vi "IMAGENES_SUB0.vi"() -> ()   [LabVIEW 2016]
uses:
  <vilib>/imath/engines/lvmath2/RunTimeEngine/BuiltInFunctions/round/NIMS_round(DBL-S).vi
  <vilib>/imath/engines/lvmath2/RunTimeEngine/NodeEndStatement/NIMS_NodeEndStatement_Output.vi
  <instcachedir>/0/NIMS_NodeEndStatement_Output_53EC0D466D134D7ABD903AC30B43404B.lvgen/NIMS_NodeEndStatement_Output_53EC0D466D134D7ABD903AC30B43404B_010.vi
  <vilib>/imath/engines/lvmath2/RunTimeEngine/ErrorHandling/NIMS_Finalize Error.vi
  <instcachedir>/0/NIMS_NodeEndStatement_Output_53EC0D466D134D7ABD903AC30B43404B.lvgen/NIMS_NodeEndStatement_Output_53EC0D466D134D7ABD903AC30B43404B_001.vi
  <vilib>/imath/engines/lvmath2/RunTimeEngine/RangeToken/NIMS_Range_R3 - Integer.vi
  <instcachedir>/0/NIMS_Range_R3 - Integer_A435E2FF893B4C718FD5055FE39FE2F6.lvgen/NIMS_Range_R3 - Integer_A435E2FF893B4C718FD5055FE39FE2F6_000.vi
  <vilib>/imath/engines/lvmath2/RunTimeEngine/CommandStatement/MC_CommandStatement_break.vi
  <vilib>/imath/engines/lvmath2/RunTimeEngine/VariableToken/NIMS_VariableToken_CondDefinedDefinedByReplace.vi
  <instcachedir>/0/NIMS_VariableToken_CondDefinedDefinedByReplace_D162CFFC24174562A9FEA619A91E1A56.lvgen/NIMS_VariableToken_CondDefinedDefinedByReplace_D162CFFC24174562A9FEA619A91E1A56_001.vi
  <vilib>/imath/engines/lvmath2/RunTimeEngine/IndexReplace/NIMS M(S,S)=S.vi
  <instcachedir>/0/NIMS M(S,S)=S_98E40400474E4398B113AE20298B4F82.lvgen/NIMS M(S,S)=S_98E40400474E4398B113AE20298B4F82_000.vi
  <vilib>/imathl/engines/lvmath/Functions/Error Handling/Create Error.vi
  <vilib>/imath/engines/lvmath2/RunTimeEngine/VariableToken/NIMS_VariableToken_CondDefined.vi
  <instcachedir>/0/NIMS_VariableToken_CondDefined_06E9DA95BD4D46A6BA55EC651A891960.lvgen/NIMS_VariableToken_CondDefined_06E9DA95BD4D46A6BA55EC651A891960_001.vi
  <vilib>/imath/engines/lvmath/Functions/Error Handling/MergeErrorsWrapper.vi
  <instcachedir>/0/NIMS_NodeEndStatement_Output_53EC0D466D134D7ABD903AC30B43404B.lvgen/NIMS_NodeEndStatement_Output_53EC0D466D134D7ABD903AC30B43404B_012.vi
panel:
  out "Anchura 2":i32
  out "Altura 2":i32
  out "Color":u32(colorbox)
  out "Anchura":i32
  out "Altura":i32
  out "IMAGEN_ORIGINAL":picture
  out "IMAGEN_MODIFICADA":picture
  out "Waveform Graph":dbl[](graph)
  in  "IMAGEN 1":path
  in  "Enum":T1(ring)
  in  "ZOOM":dbl(slide) min=0.1 max=10.0 step=0.01 scale=0.1..10.0
  in  "Desplazamiento X":dbl(slide) min=-500.0 max=500.0 step=1.0 scale=-500.0..500.0
  in  "Desplazamiento Y":dbl(slide)=500.0 min=-500.0 max=500.0 step=1.0 scale=-500.0..500.0
  in  "Giro":dbl(knob) scale=-360.0..360.0
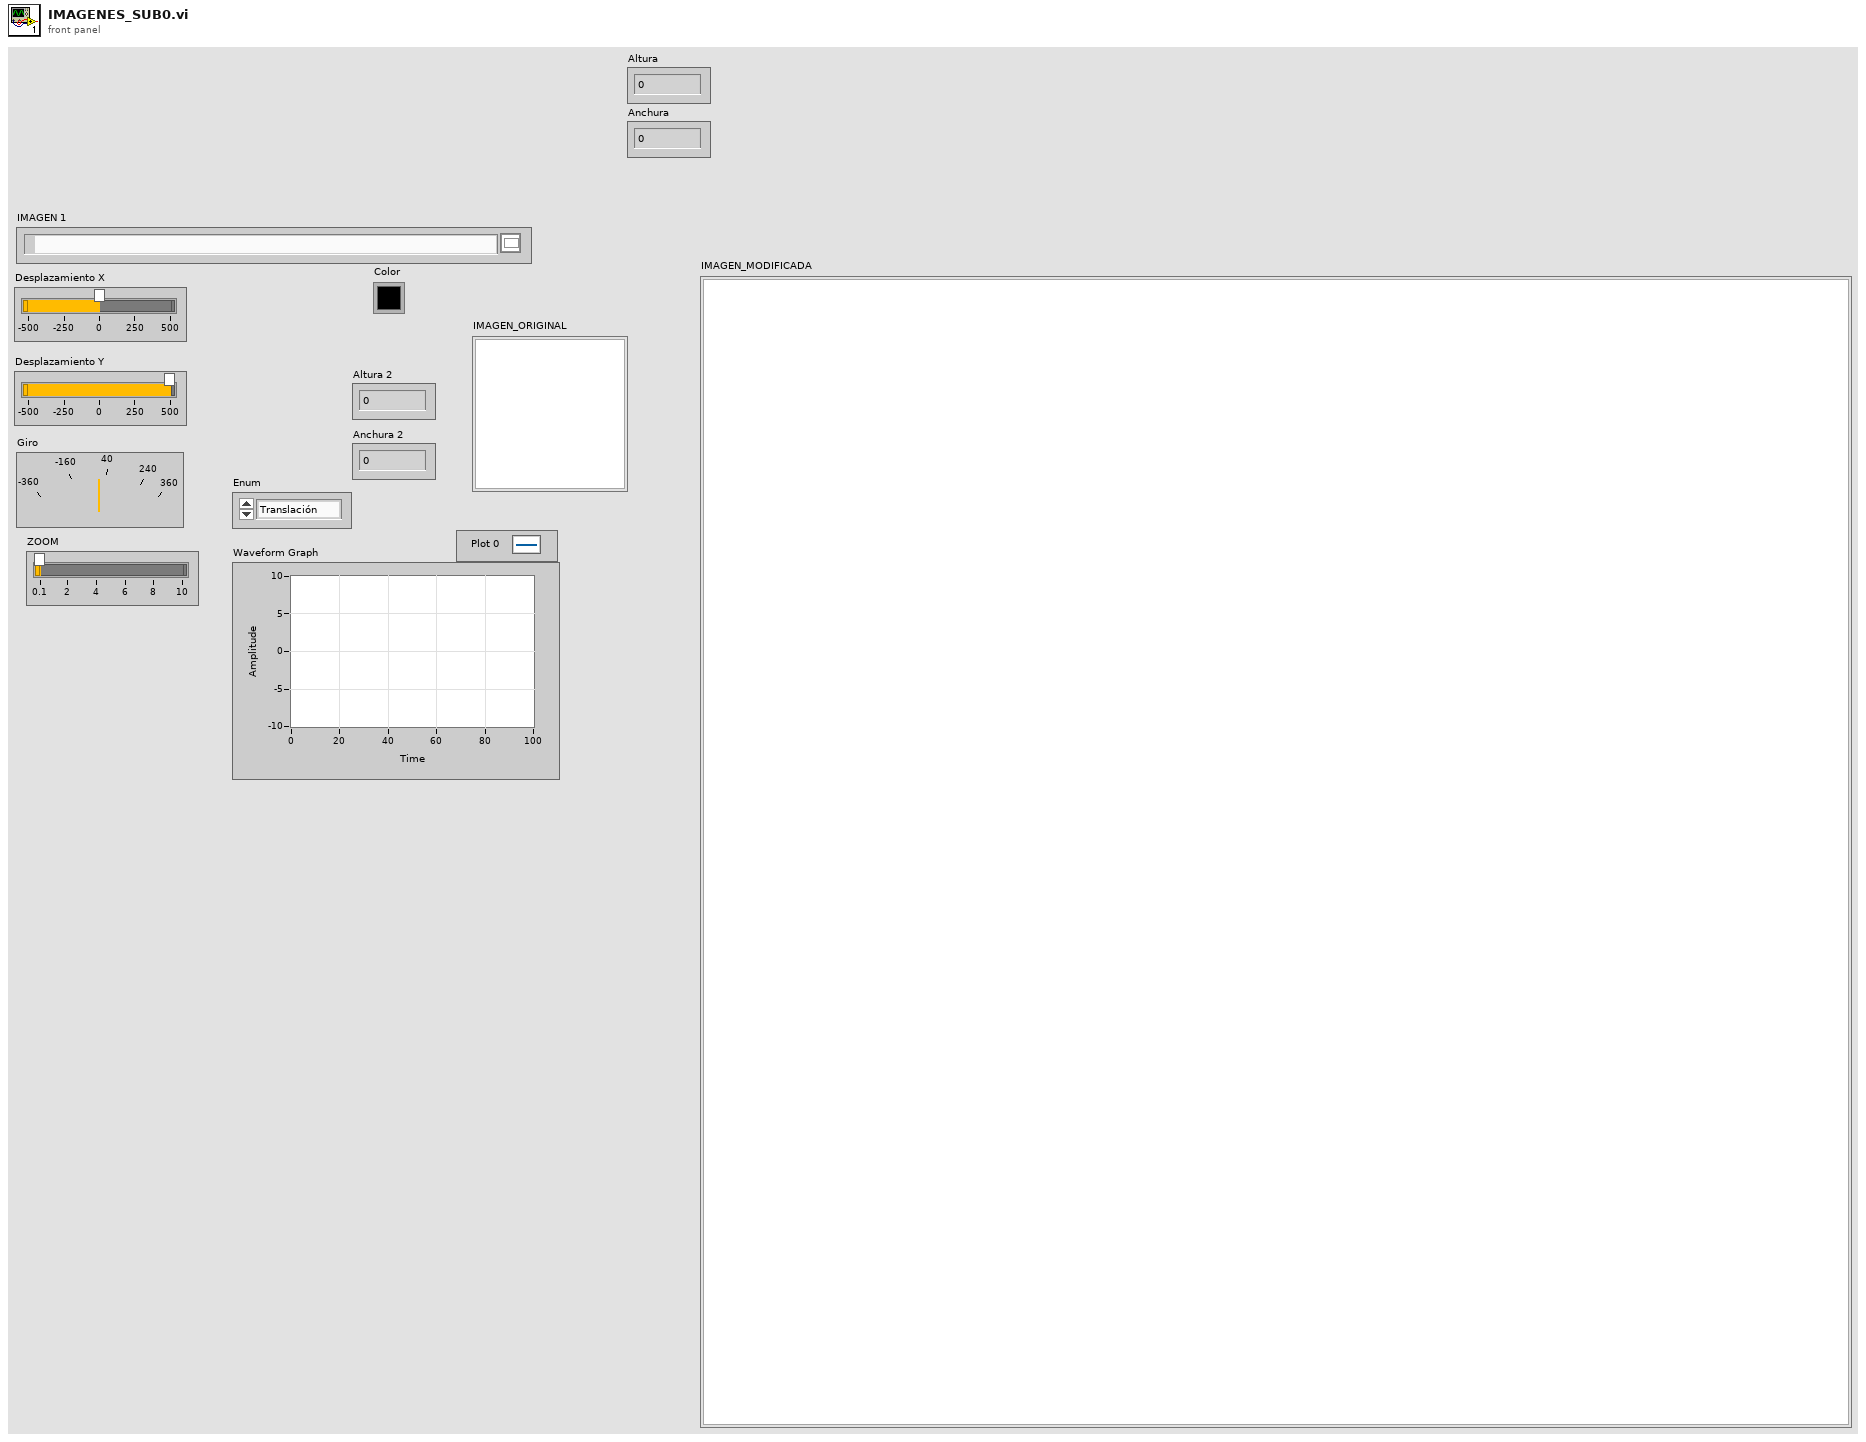
[diagram p1: front panel]
types:
  T1 = enum16{"Translación", "Rotación", "Zoom", "GIROH", "GIROV", "Sustitución", "UNION"}
  T2 = typedef "imagedata.ctl" = cluster{"image type":i32, "image depth":i32, "image":u8[], "mask":u8[], "colors":u32[], "Rectangle":cluster{"left":i16, "top":i16, "right":i16, "bottom":i16}}
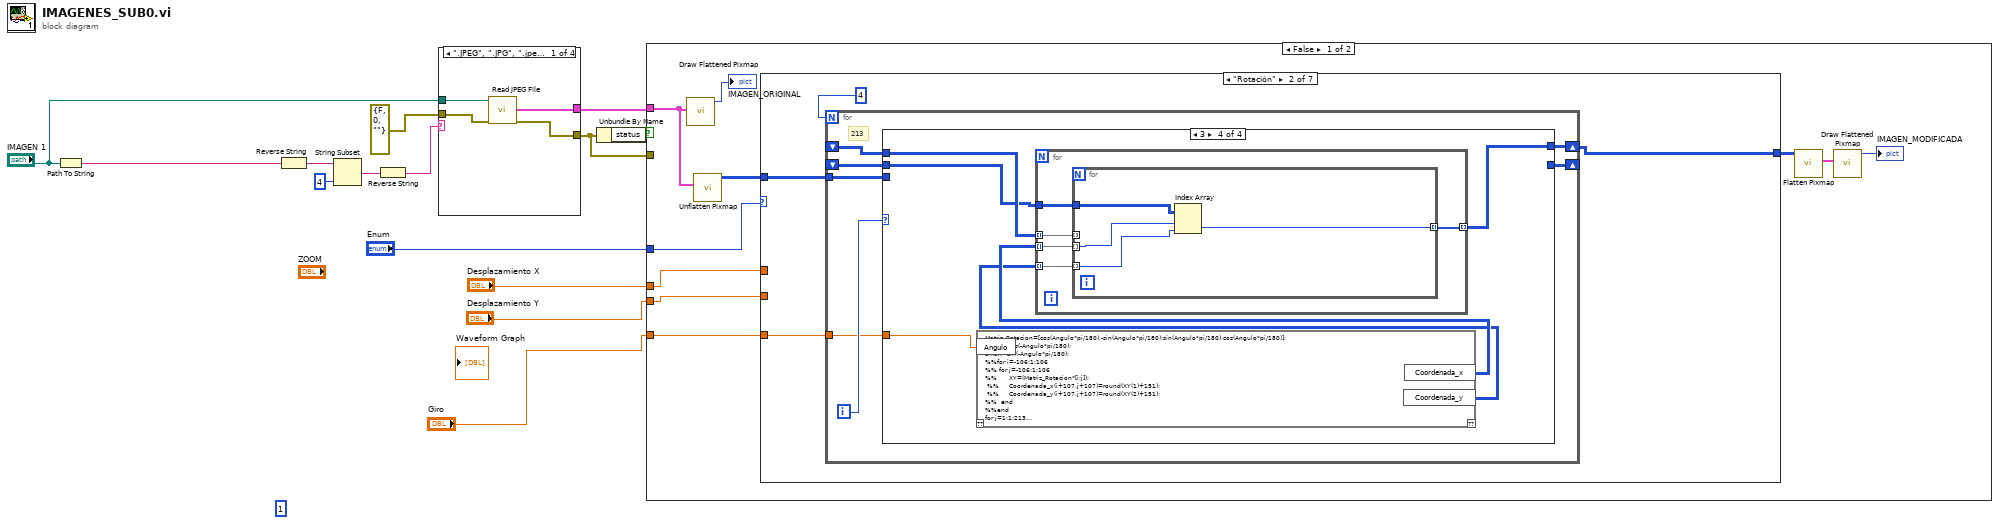
[diagram p0: block diagram]
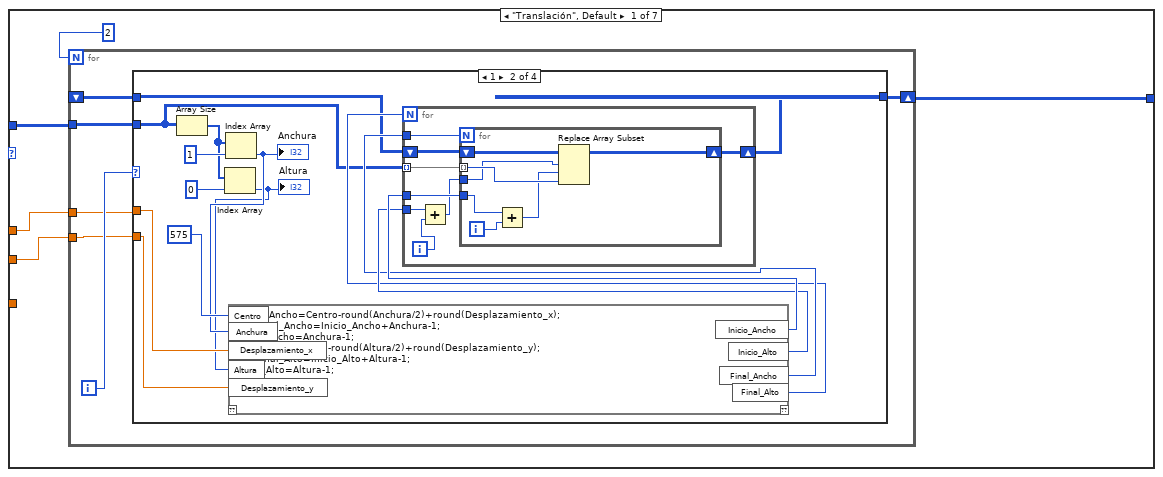
[diagram p2: hidden frame]
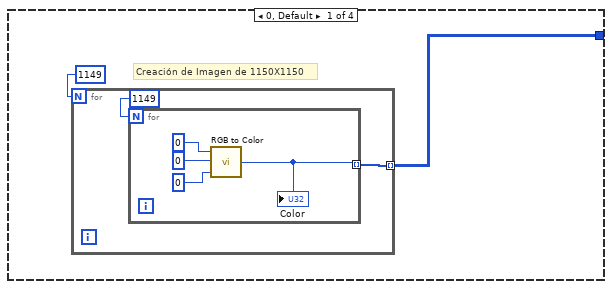
[diagram p3: hidden frame]
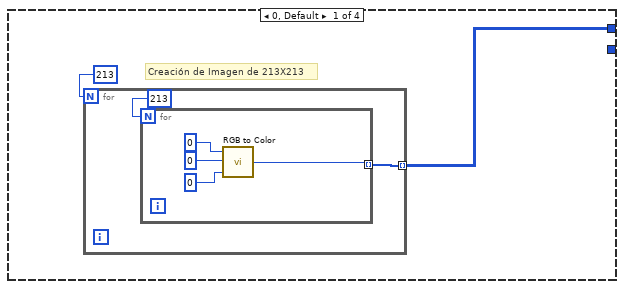
[diagram p6: hidden frame]
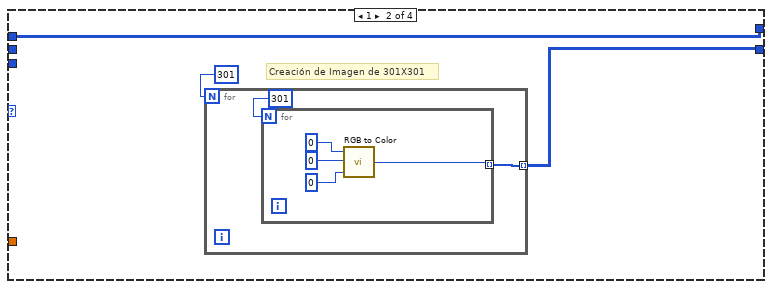
[diagram p7: hidden frame]
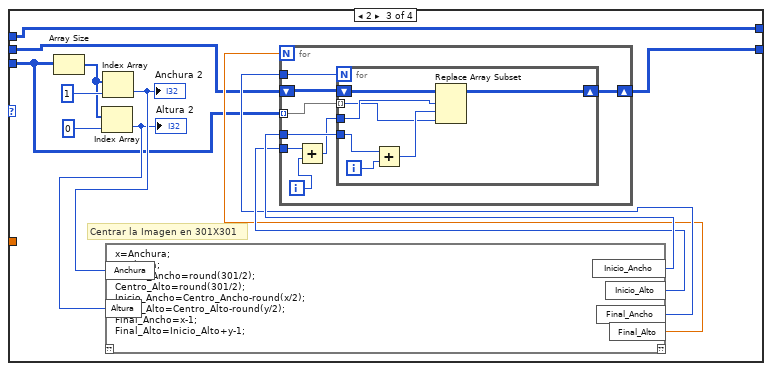
[diagram p8: hidden frame]
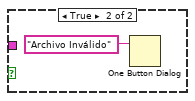
[diagram p14: hidden frame]
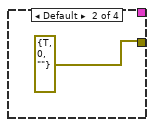
[diagram p15: hidden frame]
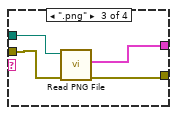
[diagram p16: hidden frame]
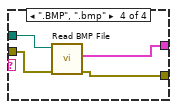
[diagram p17: hidden frame]
diagram:
  (unwired) 1
  n1 = Path To String(path="IMAGEN 1") -> (string=w14:string)
  n2 = Reverse String(1:w14) -> (0:w13:string)
  n3 = String Subset(string=w13, length (rest)=4 ("length (rest)")) -> (substring=w11:string)  [unwired: 1 in]
  n4 = Reverse String(1:w11) -> (0:w8:string)
  n5 = case shown="\".JPEG\", \".JPG\", \".jpeg\", \".jpg\"" w8 {
    tunnel: "IMAGEN 1" -> [w18 _ w23 w26]
    tunnel: errorcluster {"status"=FALSE, "code"=0, "source"=""} ("error in (no error)") -> [w17 _ w22 w25]
    tunnel: [w16 _ w21 w27] -> w7
    tunnel: [w15 errorcluster {"status"=TRUE, "code"=0, "source"=""} ("error in (no error)") w20 w24] -> w5
    frame ".JPEG", ".JPG", ".jpeg", ".jpg" {
      n6 = call <vilib>:"Read JPEG File.vi"("error in (no error)"=w17, "path to JPEG file"=w18) -> ("error out"=w15:errorcluster, "image data"=w16:T2)  [unwired: 7 in, 1 out]
    }
    frame Default {
    }
    frame ".png" {
      n7 = call <vilib>:"Read PNG File.vi"("error in (no error)"=w22, "path to PNG file"=w23) -> ("error out"=w20:errorcluster, "image data"=w21:T2)  [unwired: 7 in, 1 out]
    }
    frame ".BMP", ".bmp" {
      n8 = call <vilib>:"Read BMP File.vi"("error in (no error)"=w25, "path to BMP file"=w26) -> ("error out"=w24:errorcluster, "image data"=w27:T2)  [unwired: 7 in, 1 out]
    }
  }
  n9 = Unbundle By Name(w5) -> ("status"=w6:bool)
  n10 = case shown="False" w6 {
    tunnel: w7 -> [w36 _]
    tunnel: w5 -> [_ _]
    tunnel: "Enum" -> [w35 _]
    tunnel: "Desplazamiento X" -> [w33 _]
    tunnel: "Desplazamiento Y" -> [w32 _]
    tunnel: "Giro" -> [w28 _]
    frame False {
      n11 = call <vilib>:"Draw Flattened Pixmap.vi"("image data"=w36) -> ("new picture"=→"IMAGEN_ORIGINAL":picture)  [unwired: 8 in]
      n12 = call <vilib>:"Unflatten Pixmap.vi"("image data"=w36) -> ("24-bit pixmap"=w34:u32[][])  [unwired: 4 in, 6 out]
      n13 = case shown="\"Rotación\"" w35 {
        tunnel: w34 -> [w41 w157 _ _ _ _ _]
        tunnel: w33 -> [w40 _ _ _ _ _ _]
        tunnel: w32 -> [w39 _ _ _ _ _ _]
        tunnel: [w38 w156 _ _ _ _ _] -> w29
        tunnel: w28 -> [_ w155 _ _ _ _ _]
        frame "Translación", Default {
          n14 = for {
            N: 2 -> [_]
            shift-right: [w47] -> w38
            shift-left: _ -> [w46]
            tunnel: w41 -> [w45]
            tunnel: w40 -> [w44]
            tunnel: w39 -> [w43]
            i -> [w48]
            n15 = case shown="1" w48 {
              tunnel: [w49 w57 w153 w154] -> w47
              tunnel: w46 -> [_ w58 w153 w154]
              tunnel: w45 -> [_ w59 _ _]
              tunnel: w44 -> [_ w68 _ _]
              tunnel: w43 -> [_ w66 _ _]
              frame 0, Default {
                # "Creación de Imagen de 1150X1150"
                n16 = for {
                  N: 1149 -> [_]
                  tunnel: [w51] -> w49 mode=indexing
                  n17 = for {
                    N: 1149 -> [_]
                    tunnel: [w53] -> w51 mode=indexing
                    n18 = call <vilib>:"RGB to Color.vi"("B"=u8 0, "G"=u8 0, "R"=u8 0) -> ("Color"=w53:u32)
                    "Color" <- w53
                  }
                }
              }
              frame 1 {
                n19 = Array Size(array=w59) -> (size(s)=w69:i32[])
                n20 = Index Array(array=w69, index=0) -> (element=w64:i32)
                "Altura" <- w64
                n21 = Index Array(array=w69, index=1) -> (element=w65:i32)
                "Anchura" <- w65
                n22 = mathscript code="Inicio_Ancho=Centro-round(Anchura/2)+round(Desplazamiento_x);\n%%Final_Ancho=Inicio_Ancho+Anchura-1;\nFinal_Ancho=Anchura-1;\nInicio_Alto=Centro-round(Altura/2)+round(Desplazamiento_y);\n%%Final_Alto=Inicio_Alto+Altura-1;\nFinal_Alto=Altura-1;"("Centro"=575, "Anchura"=w65, "Desplazamiento_x"=w68, "Altura"=w64, "Desplazamiento_y"=w66) -> ("Inicio_Ancho"=w63:i32, "Inicio_Alto"=w62:i32, "Final_Ancho"=w61:i32, "Final_Alto"=w60:i32)  [unwired: 1 in, 1 out]
                n23 = for {
                  N: w60 -> [_]
                  tunnel: w63 -> [w78]
                  tunnel: w62 -> [w77]
                  tunnel: w61 -> [w75]
                  tunnel: w59 -> [w74] mode=indexing
                  shift-right: [w72] -> w57
                  shift-left: w58 -> [w73]
                  i -> [w79]
                  n24 = Add(x=w77, y=w79) -> (x+y=w76:i32)
                  n25 = for {
                    N: w75 -> [_]
                    tunnel: w78 -> [w85]
                    tunnel: w76 -> [w81]
                    tunnel: w74 -> [w82] mode=indexing
                    shift-right: [w83] -> w72
                    shift-left: w73 -> [w84]
                    i -> [w86]
                    n26 = Add(x=w85, y=w86) -> (x+y=w80:i32)
                    n27 = Replace Array Subset(array=w84, new element=w82, index (row)=w81, index (col)=w80) -> (w83:u32[][])
                  }
                }
              }
              frame 2 {
              }
              frame 3 {
              }
            }
          }
        }
        frame "Rotación" {
          n28 = for {
            N: 4 -> [_]
            shift-right: [w163] -> w156
            shift-left: _ -> [w164]
            tunnel: w157 -> [w160]
            shift-right: [w162] -> _
            shift-left: _ -> [w161]
            tunnel: w155 -> [w159]
            i -> [w165]
            # "213"
            n29 = case shown="3" w165 {
              tunnel: [w166 w175 w185 w293] -> w163
              tunnel: w164 -> [_ w175 w185 w297]
              tunnel: [_ w174 w186 _] -> w162
              tunnel: w161 -> [_ _ w184 w294]
              tunnel: w160 -> [_ _ w183 _]
              tunnel: w159 -> [_ _ _ w298]
              frame 0, Default {
                # "Creación de Imagen de 213X213"
                n30 = for {
                  N: 213 -> [_]
                  tunnel: [w168] -> w166 mode=indexing
                  n31 = for {
                    N: 213 -> [_]
                    tunnel: [w170] -> w168 mode=indexing
                    n32 = call <vilib>:"RGB to Color.vi"("B"=u8 0, "G"=u8 0, "R"=u8 0) -> ("Color"=w170:u32)
                  }
                }
              }
              frame 1 {
                # "Creación de Imagen de 301X301"
                n33 = for {
                  N: 301 -> [_]
                  tunnel: [w177] -> w174 mode=indexing
                  n34 = for {
                    N: 301 -> [_]
                    tunnel: [w179] -> w177 mode=indexing
                    n35 = call <vilib>:"RGB to Color.vi"("B"=u8 0, "G"=u8 0, "R"=u8 0) -> ("Color"=w179:u32)
                  }
                }
              }
              frame 2 {
                # "Centrar la Imagen en 301X301"
                n36 = Array Size(array=w183) -> (size(s)=w189:i32[])
                n37 = Index Array(array=w189, index=0) -> (element=w187:i32)
                "Altura 2" <- w187
                n38 = Index Array(array=w189, index=1) -> (element=w188:i32)
                "Anchura 2" <- w188
                n39 = mathscript code="x=Anchura;\ny=Altura;\nCentro_Ancho=round(301/2);\nCentro_Alto=round(301/2);\nInicio_Ancho=Centro_Ancho-round(x/2);\nInicio_Alto=Centro_Alto-round(y/2);\nFinal_Ancho=x-1;\nFinal_Alto=Inicio_Alto+y-1;"("Anchura"=w188, "Altura"=w187) -> ("Inicio_Ancho"=w193:i32, "Inicio_Alto"=w192:i32, "Final_Ancho"=w191:i32, "Final_Alto"=w190:dbl)  [unwired: 1 in, 1 out]
                n40 = for {
                  N: w190 -> [_]
                  tunnel: w193 -> [w202]
                  tunnel: w192 -> [w201]
                  tunnel: w191 -> [w199]
                  shift-right: [w197] -> w186
                  shift-left: w184 -> [w198]
                  tunnel: w183 -> [w196] mode=indexing
                  i -> [w203]
                  n41 = Add(x=w201, y=w203) -> (x+y=w200:i32)
                  n42 = for {
                    N: w199 -> [_]
                    tunnel: w202 -> [w209]
                    tunnel: w200 -> [w207]
                    shift-right: [w208] -> w197
                    shift-left: w198 -> [w205]
                    tunnel: w196 -> [w204] mode=indexing
                    i -> [w210]
                    n43 = Add(x=w209, y=w210) -> (x+y=w206:i32)
                    n44 = Replace Array Subset(array=w205, new element=w204, index (row)=w207, index (col)=w206) -> (w208:u32[][])
                  }
                }
              }
              frame 3 {
                n45 = mathscript code="Matriz_Rotacion=[cos(Angulo*pi/180),-sin(Angulo*pi/180);sin(Angulo*pi/180),cos(Angulo*pi/180)];\ncosan=cos(-Angulo*pi/180);\nsinan=sin(-Angulo*pi/180);\n%%for i=-106:1:106\n%% for j=-106:1:106\n%%      XY=(Matriz_Rotacion*[i;j]);\n %%     Coordenada_x(i+107,j+107)=round(XY(1)+151);\n %%     Coordenada_y(i+107,j+107)=round(XY(2)+151);\n%%  end\n%%end\nfor j=1:1:213\n for i=1:1:213\n       Coordenada_x(i,j)=round((i-107)*cosan-(j-107)*sinan+151);\n       Coordenada_y(i,j)=round((i-107)*sinan+(j-107)*cosan+151);\n end\nend"("Angulo"=w298) -> ("Coordenada_x"=w296:i16[][], "Coordenada_y"=w295:i16[][])  [unwired: 1 in, 1 out]
                n46 = for {
                  tunnel: w297 -> [w303] mode=indexing
                  tunnel: w296 -> [w302] mode=indexing
                  tunnel: w295 -> [w301] mode=indexing
                  tunnel: w294 -> [w300]
                  tunnel: [w299] -> w293 mode=indexing
                  n47 = for {
                    tunnel: w303 -> [_] mode=indexing
                    tunnel: w302 -> [w306] mode=indexing
                    tunnel: w301 -> [w305] mode=indexing
                    tunnel: w300 -> [w307]
                    tunnel: [w304] -> w299 mode=indexing
                    n48 = Index Array(array=w307, index (row)=w306, index (col)=w305) -> (element=w304:u32)
                  }
                }
              }
            }
          }
        }
        frame "Zoom" {
        }
        frame "GIROH" {
        }
        frame "GIROV" {
        }
        frame "Sustitución" {
        }
        frame "UNION" {
        }
      }
      n49 = call <vilib>:"Flatten Pixmap.vi"("24-bit pixmap"=w29) -> ("image data"=w30:T2)  [unwired: 10 in]
      n50 = call <vilib>:"Draw Flattened Pixmap.vi"("image data"=w30) -> ("new picture"=→"IMAGEN_MODIFICADA":picture)  [unwired: 8 in]
    }
    frame True {
      n51 = One Button Dialog(message="Archivo Inválido") -> ()  [unwired: 1 in, 1 out]
    }
  }
